vi "Transfer File.vi"(8 "error in (no error)":errorcluster) -> (0 "error out":errorcluster)   [LabVIEW 2017]
uses:
  <vilib>/WebDAVClient/NI_WebDAV.lvlib
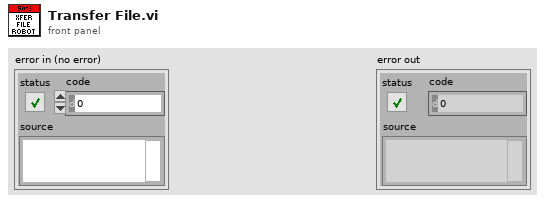
[diagram p1: front panel]
types:
  T1 = typedef "NI_WebDAV.lvlib/SessionHandle.ctl" = refnum<k1>
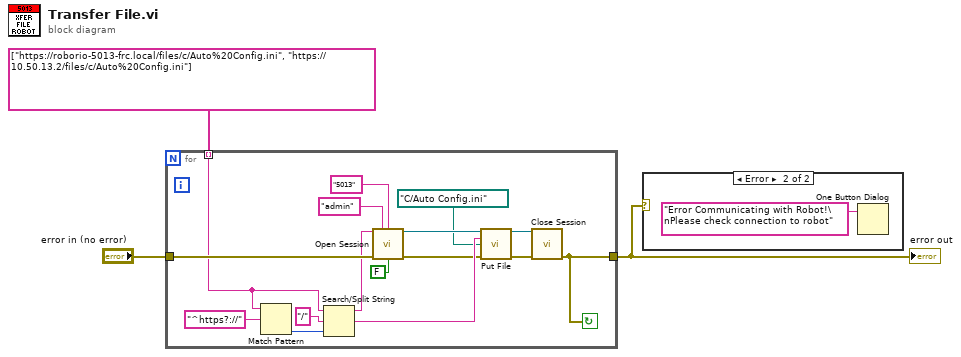
[diagram p0: block diagram]
diagram:
  n1 = for {
    tunnel: string[] ["https://roborio-5013-frc.local/files/c/Auto%20Config.ini", "https://10.50.13.2/files/c/Auto%20Config.ini"] ("file uri") -> [w12] mode=indexing
    tunnel: "error in (no error)" -> [w19]
    tunnel: [w4] -> w1
    stop <- w4 continue-if-true
    n2 = Match Pattern(string=w12, regular expression="^https?://") -> (offset past match=w18:i32)  [unwired: 1 in, 3 out]
    n3 = Search/Split String(string=w12, search string/char (-)="/", offset (0)=w18) -> (substring before match=w15:string, match + rest of string=w7:string)  [unwired: 1 out]
    n4 = call <vilib>:"Open Session.vi"("host uri prefix"=w15, "username"="admin", "password"="5013", "error in (no error)"=w19, "verify server?"=FALSE) -> ("session handle out"=w8:T1, "error out"=w6:errorcluster)  [unwired: 9 in]
    n5 = call <vilib>:"Put File.vi"("session handle"=w8, "relative uri"=w7, "local file path"=path "C:/Auto Config.ini" ("Path (dialog)"), "error in (no error)"=w6) -> ("session handle out"=w10:T1, "error out"=w9:errorcluster)  [unwired: 9 in, 1 out]
    n6 = call <vilib>:"Close Session.vi"("session handle"=w10, "error in (no error)"=w9) -> ("error out"=w4:errorcluster)  [unwired: 13 in]
  }
  "error out" <- w1
  n7 = case shown="Error" w1 {
    frame No Error {
    }
    frame Error {
      n8 = One Button Dialog(message="Error Communicating with Robot!\nPlease check connection to robot") -> ()  [unwired: 1 in, 1 out]
    }
  }
